vi "Swap (No Check).vi"(8 "error in (no error)":errorcluster, 9 "size":u64 format="%d bytes", 10 "Pointer y":refnum<class "Pointer.lvclass">, 11 "Pointer x":refnum<class "Pointer.lvclass">) -> (0 "error out":errorcluster, 2 "Pointer y":refnum<class "Pointer.lvclass">, 3 "Pointer x":refnum<class "Pointer.lvclass">)   [LabVIEW 2027, in "Memory Manager.lvlib" / "Pointer.lvclass"]
doc: "Swaps <b>size</b> bytes between the sections of memory referred to by the two provided <b>Pointers</b>. The source and destination memory blocks should not overlap.\n\n<b>Note:</b> This VI is <b>unsafe</b>, meaning it does not performs null pointer and bounds checks to prevent invaid memory access. Invalid arguments provided to this method can crash or corrupt LabVIEW memory."
uses:
  Pointer.lvclass
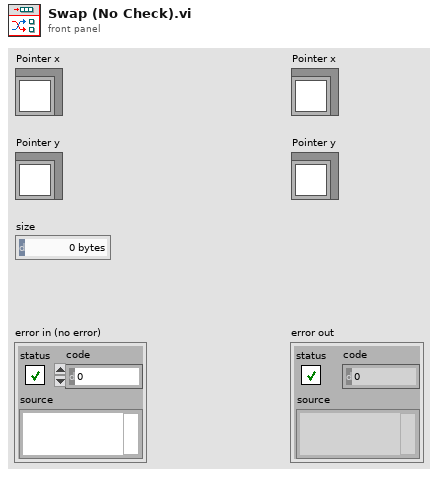
[diagram p1: front panel]
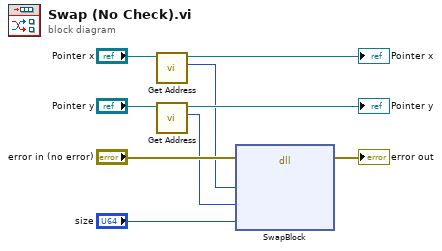
[diagram p0: block diagram]
diagram:
  n1 = call "Get Address.vi"("Pointer in"="Pointer x") -> ("address"=w3:u64, "Pointer out"=→"Pointer x":refnum<class "Pointer.lvclass">)  [unwired: 9 in]
  n2 = call "Get Address.vi"("Pointer in"="Pointer y") -> ("address"=w2:u64, "Pointer out"=→"Pointer y":refnum<class "Pointer.lvclass">)  [unwired: 9 in]
  n3 = dll-call lib="LabVIEW" fn="SwapBlock"(error in="error in (no error)", "src"=w3, "dst"=w2, "size"="size") -> (error out=→"error out":errorcluster)  [unwired: 6 in, 1 out]
